vi "SetByteOrder.vi"(8 "error in (no error)":errorcluster, 10 "byte order (0:big-endian, network order)":T1(ring), 11 "All_In_One in":refnum<class "AllInOne.lvclass">) -> (0 "error out":errorcluster, 3 "All_In_One out":refnum<class "AllInOne.lvclass">)   [LabVIEW 2020, in "AllInOne.lvclass"]
uses:
  AllInOne.lvclass
  AllInOne.lvclass/AllInOne.ctl
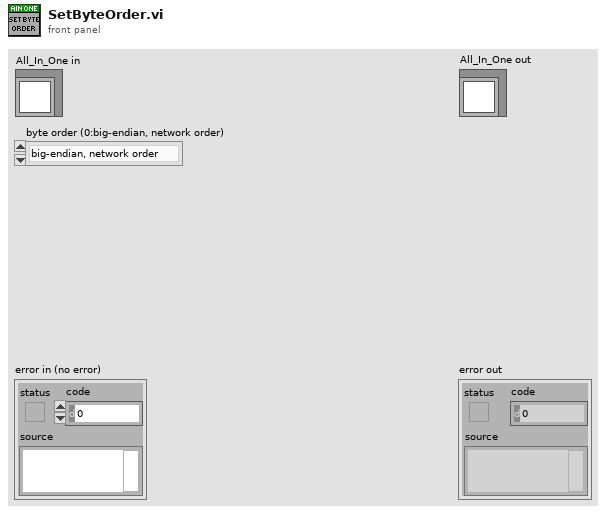
[diagram p1: front panel]
types:
  T1 = enum16{"big-endian, network order", "native, host order", "little-endian"}
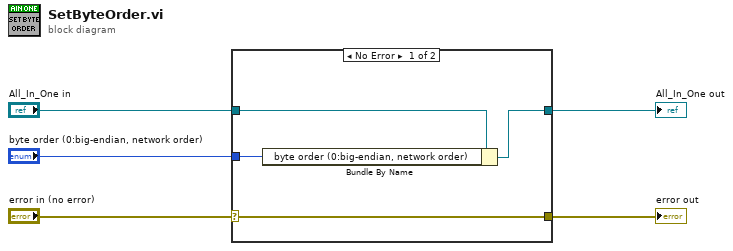
[diagram p0: block diagram]
diagram:
  n1 = case shown="No Error" "error in (no error)" {
    selector: "error in (no error)" -> [w9 w11]
    tunnel: [w9 w11] -> w4
    tunnel: "All_In_One in" -> [w8 w10]
    tunnel: [w7 w10] -> w2
    tunnel: "byte order (0:big-endian, network order)" -> [w6 _]
    frame No Error {
      n2 = Bundle By Name(cluster=w8, "byte order (0:big-endian, network order)"=w6) -> (w7:refnum<class "AllInOne.lvclass">)
    }
    frame Error {
    }
  }
  "error out" <- w4
  "All_In_One out" <- w2
